vi "Determine_Data_SubVI.vi"() -> ()   [LabVIEW 2014]
panel:
  out "Output Value":dbl
  in  "SO2":string
  in  "Ozone":string
  in  "CO":string
  in  "FGGA":string
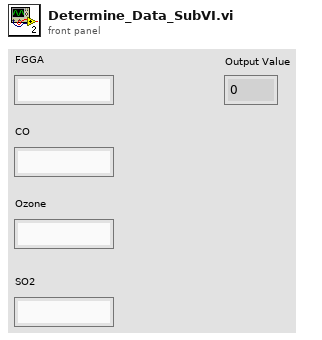
[diagram p1: front panel]
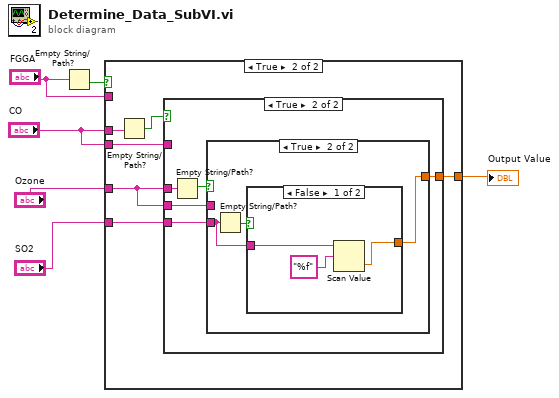
[diagram p0: block diagram]
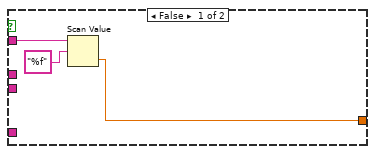
[diagram p2: hidden frame]
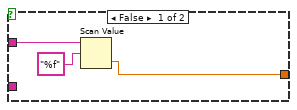
[diagram p3: hidden frame]
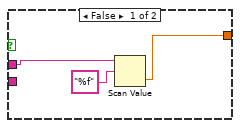
[diagram p4: hidden frame]
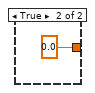
[diagram p5: hidden frame]
diagram:
  n1 = Empty String/Path?(string/path="FGGA") -> (empty?=w6:bool)
  n2 = case shown="True" w6 {
    tunnel: "FGGA" -> [w8 _]
    tunnel: [w7 w12] -> w4
    tunnel: "CO" -> [_ w15]
    tunnel: "CO" -> [_ w13]
    tunnel: "Ozone" -> [_ w10]
    tunnel: "SO2" -> [_ w11]
    frame False {
      n3 = Scan Value(string=w8, format string="%f") -> (value=w7:dbl)  [unwired: 1 in, 1 out]
    }
    frame True {
      n4 = Empty String/Path?(string/path=w15) -> (empty?=w14:bool)
      n5 = case shown="True" w14 {
        tunnel: w13 -> [w17 _]
        tunnel: w10 -> [_ w23]
        tunnel: [w16 w19] -> w12
        tunnel: w11 -> [_ w21]
        tunnel: w10 -> [_ w20]
        frame False {
          n6 = Scan Value(string=w17, format string="%f") -> (value=w16:dbl)  [unwired: 1 in, 1 out]
        }
        frame True {
          n7 = Empty String/Path?(string/path=w23) -> (empty?=w22:bool)
          n8 = case shown="True" w22 {
            tunnel: w21 -> [_ w27]
            tunnel: w20 -> [w25 _]
            tunnel: [w24 w28] -> w19
            frame False {
              n9 = Scan Value(string=w25, format string="%f") -> (value=w24:dbl)  [unwired: 1 in, 1 out]
            }
            frame True {
              n10 = Empty String/Path?(string/path=w27) -> (empty?=w29:bool)
              n11 = case shown="False" w29 {
                tunnel: [w30 0.0] -> w28
                tunnel: w27 -> [w31 _]
                frame False {
                  n12 = Scan Value(string=w31, format string="%f") -> (value=w30:dbl)  [unwired: 1 in, 1 out]
                }
                frame True {
                }
              }
            }
          }
        }
      }
    }
  }
  "Output Value" <- w4
